vi "Analyze Segments.vi"(8 "error in (no error)":errorcluster, 11 "VISA resource name":refnum<visa-resource-name>) -> (0 "error out":errorcluster, 3 "VISA resource name out":refnum<visa-resource-name>)   [LabVIEW 2010, in "Agilent 2000 3000 X-Series.lvlib"]
doc: "Calculates measurement statistics and/or infinite persistence over all segments that have been acquired.\n\n<B>Note(s):</B>\n(1) The oscilloscope must be stopped and in segmented acquisition mode with <B>Configure Acquisition.vi</B>, with either quick measurements or infinite persistence on.\n(2) This operation is available when the segmented memory option (Option SGM) is enabled."
uses:
  <instrlib>/Agilent 2000 3000 X-Series/Agilent 2000 3000 X-Series.lvlib
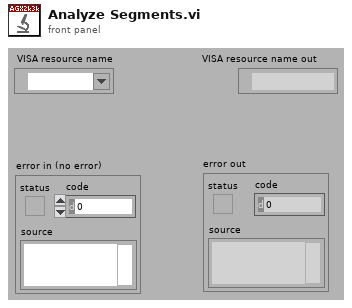
[diagram p1: front panel]
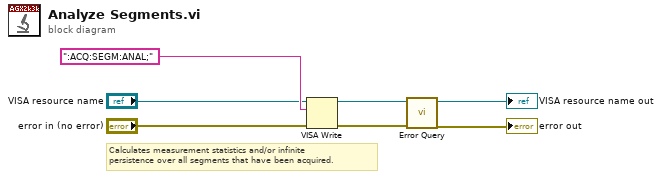
[diagram p0: block diagram]
diagram:
  # "Calculates measurement statistics and/or infinite \npersistence over all segments that have been acquired."
  n1 = VISA Write(VISA resource name="VISA resource name", write buffer=":ACQ:SEGM:ANAL;", error in (no error)="error in (no error)") -> (VISA resource name out=w4:refnum<visa-resource-name>, error out=w3:errorcluster)  [unwired: 1 out]
  n2 = call <instrlib>:"Error Query.vi"("error in (no error)"=w3, "VISA resource name"=w4) -> ("error out"=→"error out":errorcluster, "VISA resource name out"=→"VISA resource name out":refnum<visa-resource-name>)  [unwired: 8 out]
